vi "IMS Stepper Command.vi"(0 "Instrument Address":refnum<visa-resource-name>, 1 "Motor Number":u32=1 min=1 max=255 step=1, 2 "Command":string, 3 "Mode":bool, 4 "Timeout Limit":sgl=0.1 format="%.2f", 5 "error in (no error)":errorcluster) -> (6 "Timeout":bool, 7 "Response":string, 8 "error out":errorcluster)   [LabVIEW 2018]
uses:
  Serial Support VISA.llb/Serial Actions.ctl
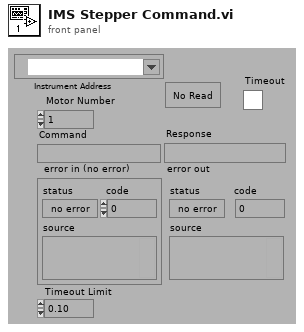
[diagram p1: front panel]
types:
  T1 = typedef "Serial Actions.ctl" = enum16{"Init", "Break", "Clear Buffer", "Write", "Read", "N Bytes", "Lock", "Unlock", "Close"}
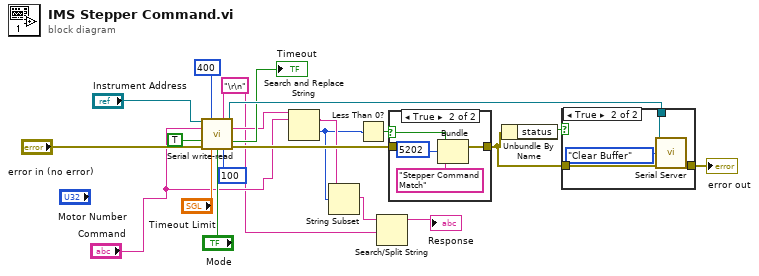
[diagram p0: block diagram]
diagram:
  w1 = "\r\n" ("EOT Chars (cr/lf)")
  n1 = call "Serial write-read.vi"("VISA Resource Name"="Instrument Address", "Max Char to Read"=u32 400, "EOT Chars (cr/lf)"=w1, "String To Send"="Command", "Clear Buffer?"=TRUE, "error in (no error)"="error in (no error)", "Timeout Limit"="Timeout Limit", "Read Echo?"="Mode", "milliseconds to wait"=u32 100) -> ("dup VISA Resource Name"=w15:refnum<visa-resource-name>, "Serial Read"=w8:string, "Timeout"=→"Timeout":bool, "error out"=w19:errorcluster)  [unwired: 1 in, 2 out]
  n2 = Search and Replace String(input string=w8, search string="Command") -> (result string=w4:string, offset past replacement=w3:i32)  [unwired: 6 in, 2 out]
  n3 = String Subset(string=w4, offset (0)=w3) -> (substring=w5:string)  [unwired: 1 in]
  n4 = Less Than 0?(x=w3) -> (x < 0?=w6:bool)
  n5 = Search/Split String(string=w5, search string/char (-)=w1) -> (substring before match=→"Response":string)  [unwired: 1 in, 2 out]
  n6 = case shown="True" w6 {
    selector: w6 -> [_ w25]
    tunnel: [w22 w26] -> w10
    tunnel: w19 -> [w22 _]
    frame False {
    }
    frame True {
      n7 = Bundle(w25, 5202, "Stepper Command Match") -> (w26:errorcluster)  [unwired: 1 in]
    }
  }
  n8 = Unbundle By Name(w10) -> ("status"=w20:bool)
  n9 = case shown="True" w20 {
    tunnel: w15 -> [_ w30]
    tunnel: [w27 w29] -> w11
    tunnel: w10 -> [w27 w28]
    frame False {
    }
    frame True {
      n10 = call "Serial Server.vi"("VISA Resource Name"=w30, "Action"=Serial_Actions."Clear Buffer", "error in (no error)"=w28) -> ("error out"=w29:errorcluster)  [unwired: 8 in, 4 out]
    }
  }
  "error out" <- w11
